vi "VL53L0X_SetDeviceMode.vi"(11 "REV2mDistanceSensorDevRef":T1) -> (3 "REV2mDistanceSensorDevRef Out":T1)   [LabVIEW 2019, in "DistanceSensorDriver.lvlib"]
uses:
  DistanceSensorDriver.lvlib
  Typedef/REV2mDistanceSensorDevRef.ctl
  Typedef/Ports.ctl
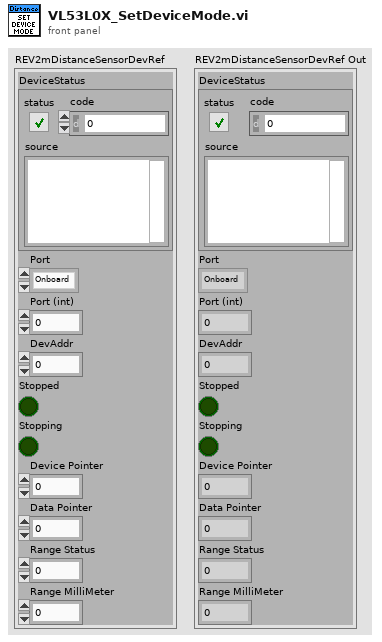
[diagram p1: front panel]
types:
  T1 = typedef "DistanceSensorDriver.lvlib/REV2mDistanceSensorDevRef.ctl" = cluster{"DeviceStatus":errorcluster, "Port":T2, "Port (int)":i32, "DevAddr":i32, "Stopped":bool, "Stopping":bool, "Device Pointer":u64, "Data Pointer":u64, "Range Status":u8, "Range MilliMeter":u16}
  T2 = typedef "DistanceSensorDriver.lvlib/Ports.ctl" = enum32{"Onboard", "MXP"}
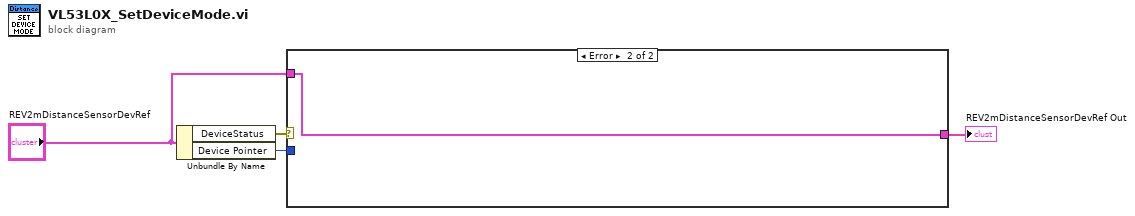
[diagram p0: block diagram]
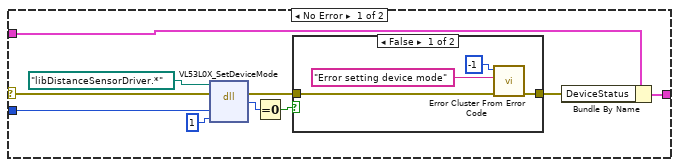
[diagram p2: hidden frame]
diagram:
  n1 = Unbundle By Name("REV2mDistanceSensorDevRef") -> ("DeviceStatus"=w1:errorcluster, "Device Pointer"=w4:u64)
  n2 = case shown="Error" w1 {
    selector: w1 -> [w5 _]
    tunnel: w4 -> [w9 _]
    tunnel: [w8 w20] -> w3
    tunnel: "REV2mDistanceSensorDevRef" -> [w7 w20]
    frame No Error {
      n3 = dll-call lib="?" fn="VL53L0X_SetDeviceMode"(path in=path "libDistanceSensorDriver.*", error in=w5, "Dev"=w9, "DeviceMode"=u8 1) -> (error out=w10:errorcluster, "Status"=w11:i32)  [unwired: 3 in, 1 out]
      n4 = Equal To 0?(x=w11) -> (x = 0?=w14:bool)
      n5 = case shown="False" w14 {
        tunnel: w10 -> [w15 w19]
        tunnel: [w18 w19] -> w13
        frame False {
          n6 = call <vilib>:"Error Cluster From Error Code.vi"("error in (no error)"=w15, "error message (\"\")"="Error setting device mode" ("error message (\"\")"), "error code (0)"=-1) -> ("error out"=w18:errorcluster)  [unwired: 6 in]
        }
        frame True {
        }
      }
      n7 = Bundle By Name(cluster=w7, "DeviceStatus"=w13) -> (w8:T1)
    }
    frame Error {
    }
  }
  "REV2mDistanceSensorDevRef Out" <- w3
